vi "Timer.vi"(8 "error in (no error)":errorcluster, 9 "Command":enum16{"Reset", "Get Time", "Check Time"}(ring), 10 "Wait Time (s)":dbl) -> (0 "error out":errorcluster, 1 "Elapsed Time (s)":dbl, 2 "Time Expired?":bool)   [LabVIEW 2010]
doc: "This VI functions as a functional global for timing. This VI serves as a stop watch/timer depending on the application.\n\nInputs:\nWait Time - (Timer mode) Time to wait\nCommand - Reset -> Resets the timer with current time value\n Get Time -> Gets time elapsed since last reset (stop watch mode)\n Check Time -> Compares time elapse since last reset with wait time value.\n Time expired? = T if required amount of time has passed.\n\nOutputs:\nTime Expired? - True if time specified has passed since last reset (timer mode only)\nElapsed Time (s) - Time elapsed since last reset (seconds)"
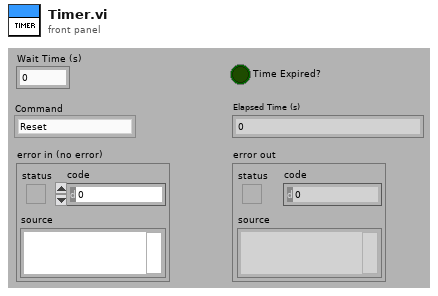
[diagram p1: front panel]
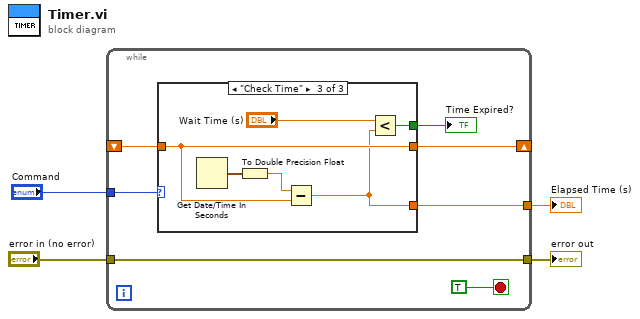
[diagram p0: block diagram]
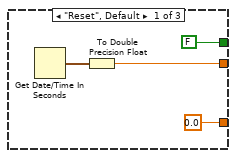
[diagram p2: hidden frame]
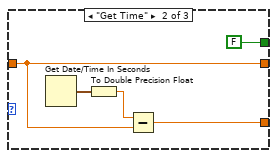
[diagram p3: hidden frame]
diagram:
  n1 = while {
    tunnel: "Command" -> [w11]
    tunnel: [w8] -> w3
    shift-right: [w9] -> _
    shift-left: _ -> [w7]
    tunnel: [w5] -> w2
    tunnel: "error in (no error)" -> [w5]
    stop <- TRUE stop-if-true
    n2 = case shown="\"Check Time\"" w11 {
      tunnel: [0.0 w19 w21] -> w8
      tunnel: [w15 w16 w24] -> w9
      tunnel: w7 -> [_ w16 w24]
      tunnel: [FALSE FALSE w23] -> w6
      frame "Reset", Default {
        n3 = Get Date/Time In Seconds() -> (seconds since 1Jan1904=w14:timestamp)
        n4 = To Double Precision Float(number=w14) -> (double precision float=w15:dbl)
      }
      frame "Get Time" {
        n5 = Get Date/Time In Seconds() -> (seconds since 1Jan1904=w20:timestamp)
        n6 = To Double Precision Float(number=w20) -> (double precision float=w18:dbl)
        n7 = Subtract(x=w18, y=w16) -> (x-y=w19:dbl)
      }
      frame "Check Time" {
        n8 = Get Date/Time In Seconds() -> (seconds since 1Jan1904=w26:timestamp)
        n9 = To Double Precision Float(number=w26) -> (double precision float=w25:dbl)
        n10 = Subtract(x=w25, y=w24) -> (x-y=w21:dbl)
        n11 = Less?(x="Wait Time (s)", y=w21) -> (x < y?=w23:bool)
      }
    }
    "Time Expired?" <- w6
  }
  "Elapsed Time (s)" <- w3
  "error out" <- w2
